vi "Plugin-001-MaterialTest.vi"(0 "Configuration Page":refnum<class "Material-ConfigPage.lvclass">, 11 "error in":errorcluster) -> (15 "error out":errorcluster)   [LabVIEW 2013, in "Material-RunTest.lvclass"]
doc: "DisplayName=\"Deploy Configuration Template\"\nDescription=\"This VI serves as a template page for the Deploy Configuration UI.\""
uses:
  Plugins/Run Material Test/Material-RunTest.lvclass
  Reuse Library/featherweight/Core/Sequencer/FTW-Sequencer.lvclass
  Reuse Library/featherweight/Core/Messaging/Message.Actor/FTW-Message-Actor.lvclass
  Material-ConfigPage.lvclass
  <vilib>/Utility/miscctls.llb/LVPointTypeDef.ctl
  Plugins/Motion Control/Motion-ControlAll.lvclass
  <instrlib>/Keyence LK-G5000/Keyence LK-G5000.lvlib
  Reuse Library/Database API/Database-API.lvclass
  <vilib>/addons/_LabVIEW Style Book/Utilities/Style Book Utilities.lvlib
  <vilib>/ErrorRing/Error Ring.xnode
  <vilib>/Utility/error.llb/Error Cluster From Error Code.vi
panel:
  in  "Find Home Position":bool
  out "Average Thickness Line 3":dbl format="%_5g"
  out "Line 3 test passed?":bool
  out "Line 3 Measurement Graph":dbl[](graph)
  out "Average Thickness Line 2":dbl format="%_5g"
  out "Line 2 test passed?":bool
  out "Line 2 Measurement Graph":dbl[](graph)
  out "Average Thickness Line 1":dbl format="%_5g"
  out "Line 1 test passed?":bool
  out "Line 1 Measurement Graph":dbl[](graph)
  in  "Zero Laser":bool
  in  "Stop Button":bool
  out "Overall Sheet Passed?":bool
  out "Total Average Thickness of Sheet":dbl format="%_6g"
  out "Thickness Measured Real Time":dbl format="%_6g"
  in  "Begin Test":bool
  out "Message Received":string
  # "Settings"
  # "Inputs"
  # "Outputs"
  # "First Plugin"
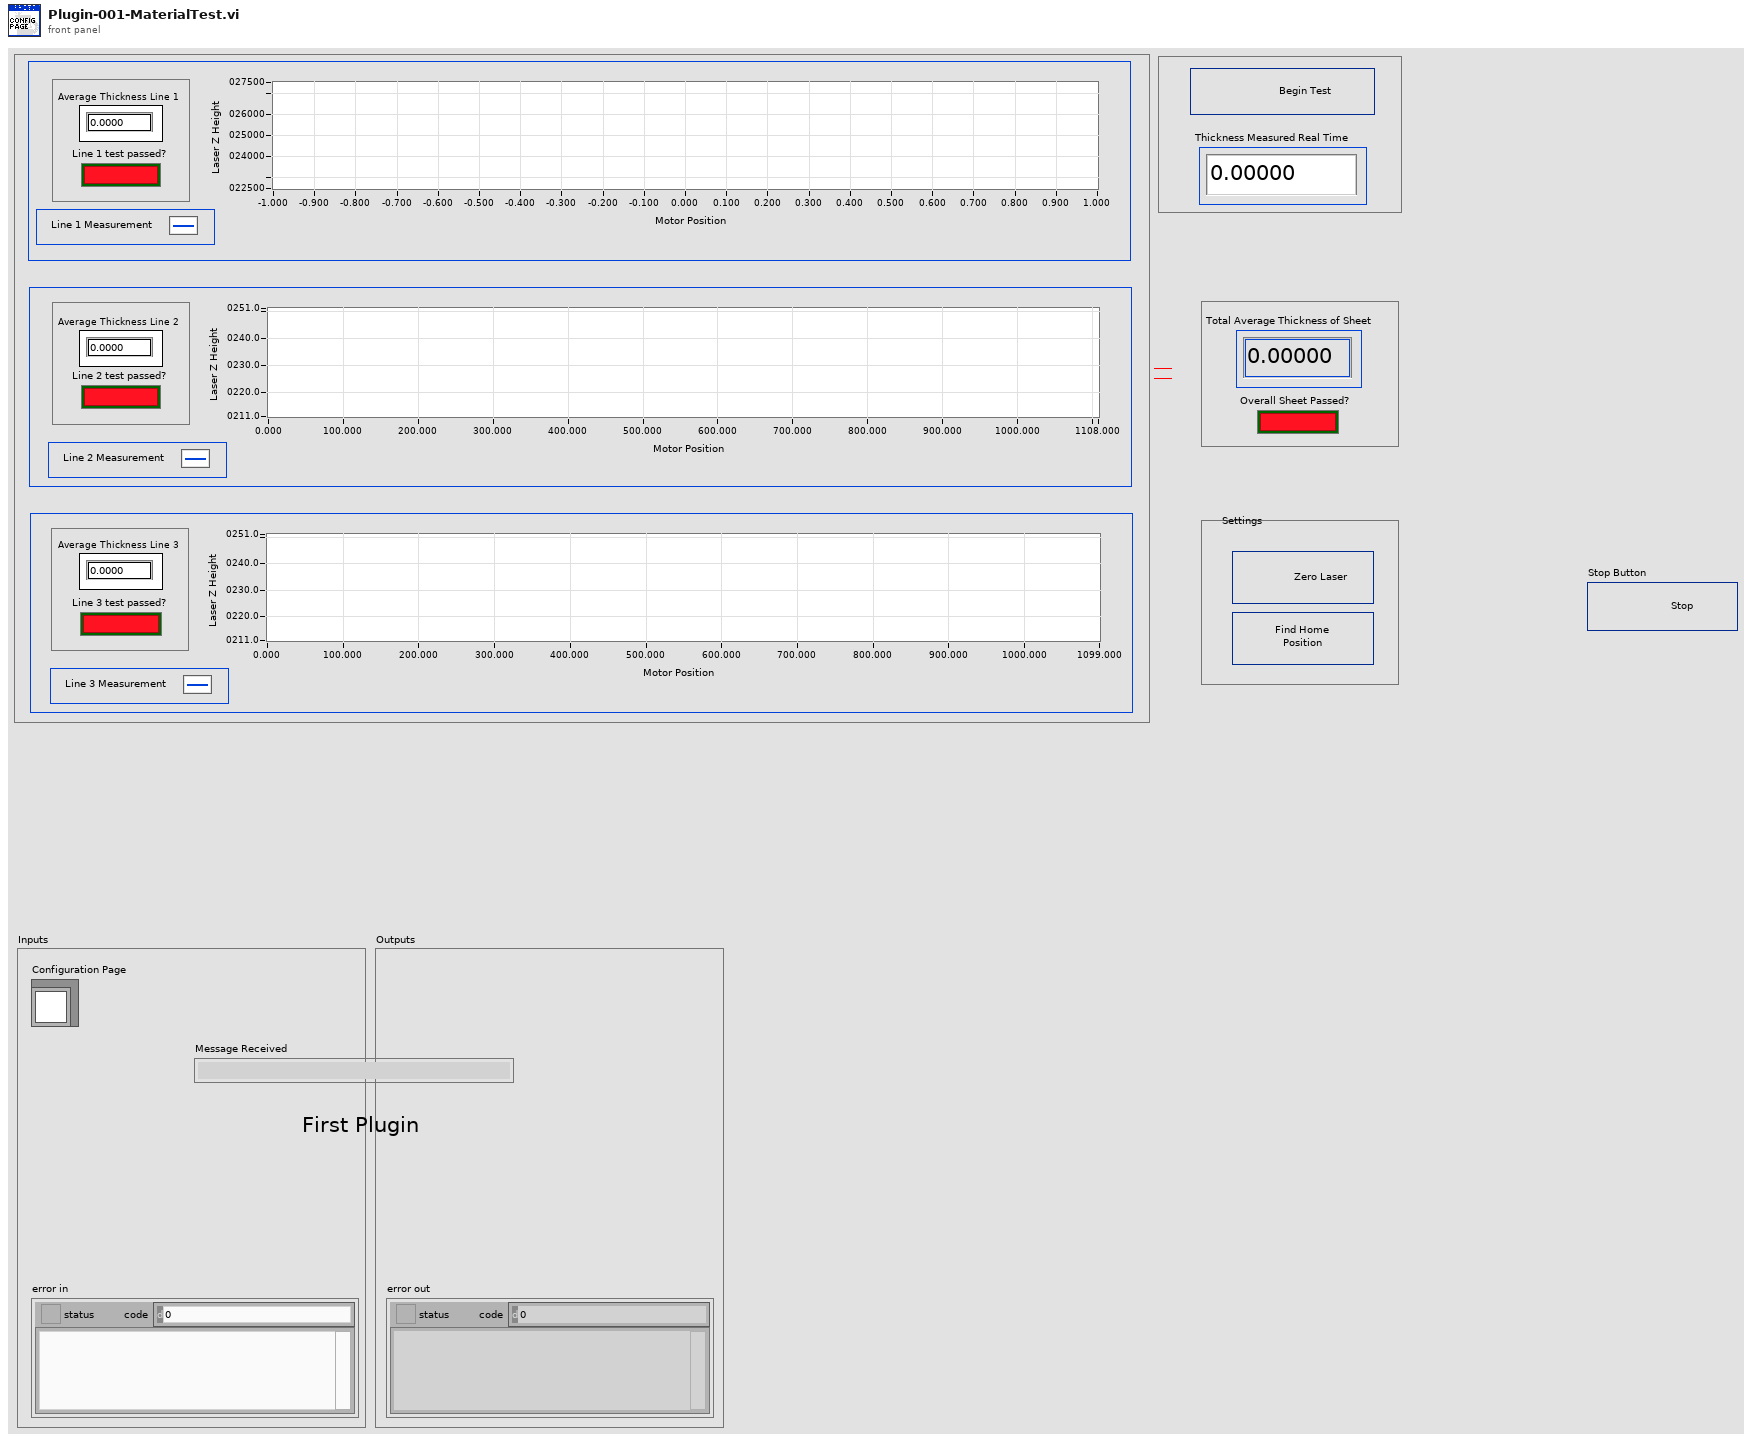
[diagram p1: front panel]
types:
  T1 = enum8{"Enabled", "Disabled", "Disabled and Grayed Out"}
  T2 = typedef "LVPointTypeDef.ctl" = cluster{"Horizontal":i16, "Vertical":i16}
  T3 = cluster{"PageCommands":refnum<event-registration>}
  T4 = cluster{"Zero Button Pressed":bool, "Home Button Pressed":bool}
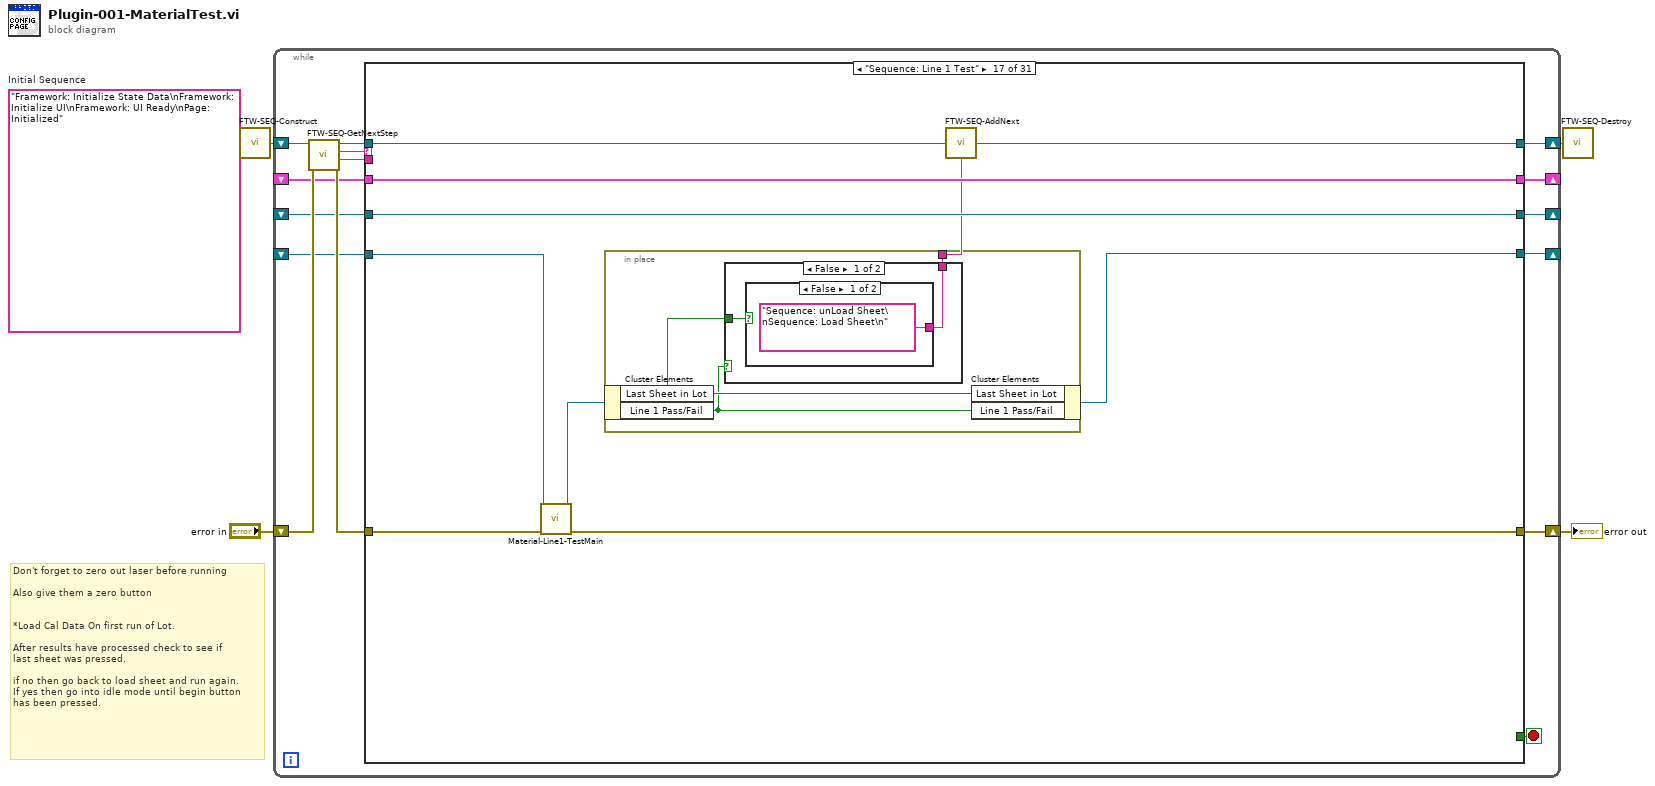
[diagram p0: block diagram]
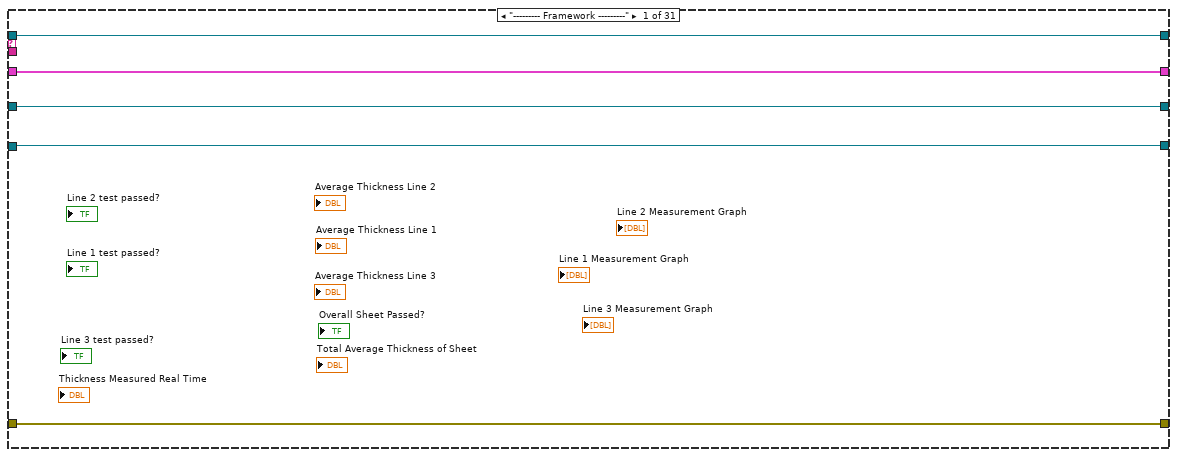
[diagram p2: hidden frame]
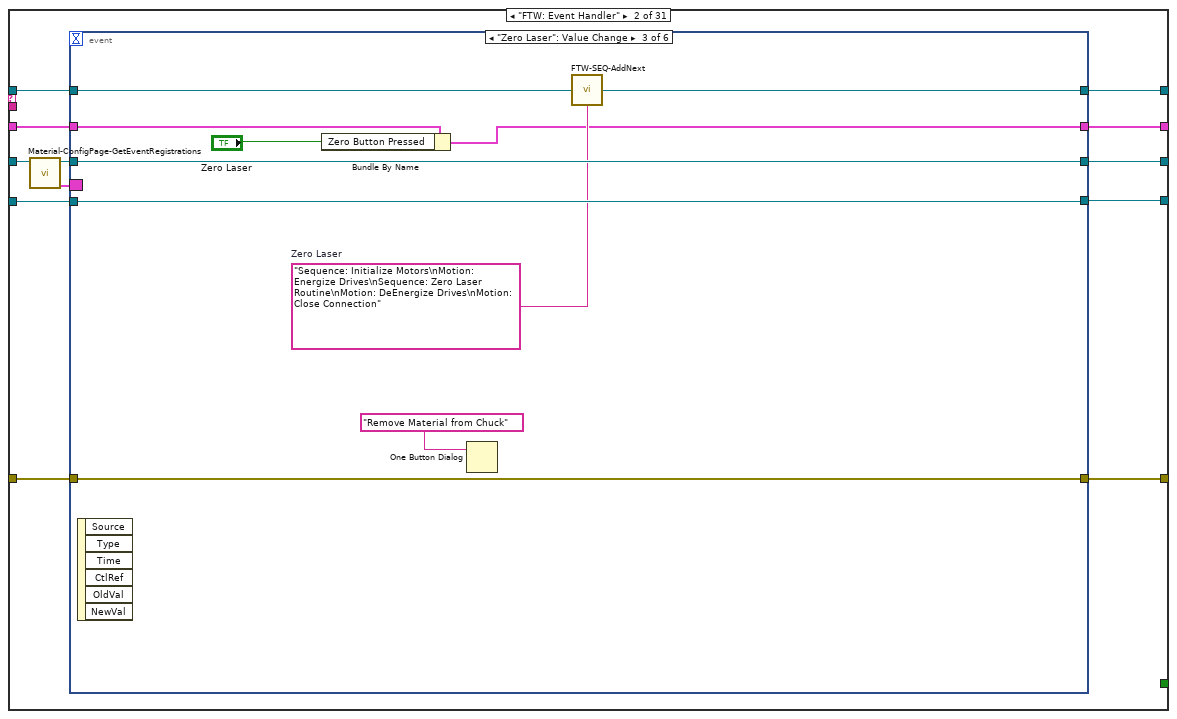
[diagram p3: hidden frame]
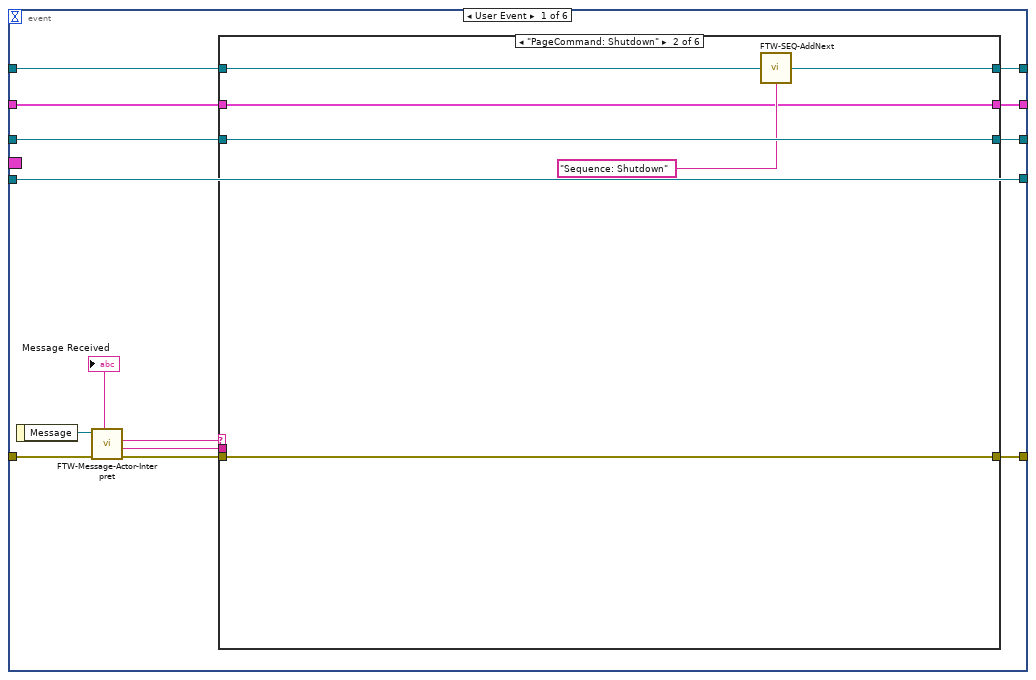
[diagram p4: hidden frame]
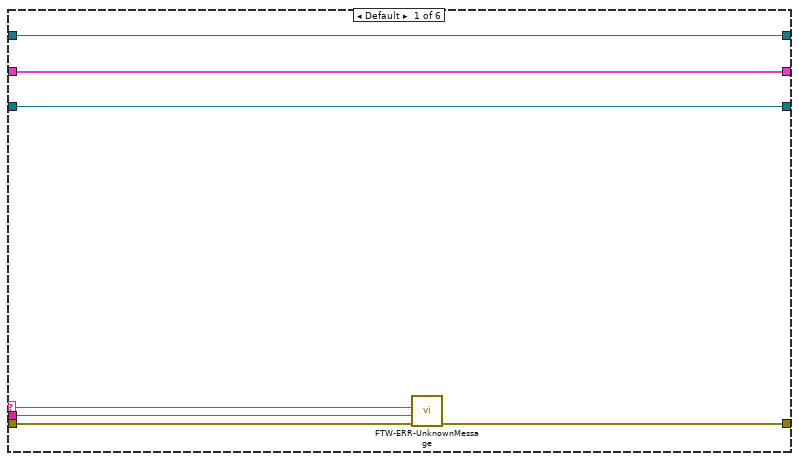
[diagram p5: hidden frame]
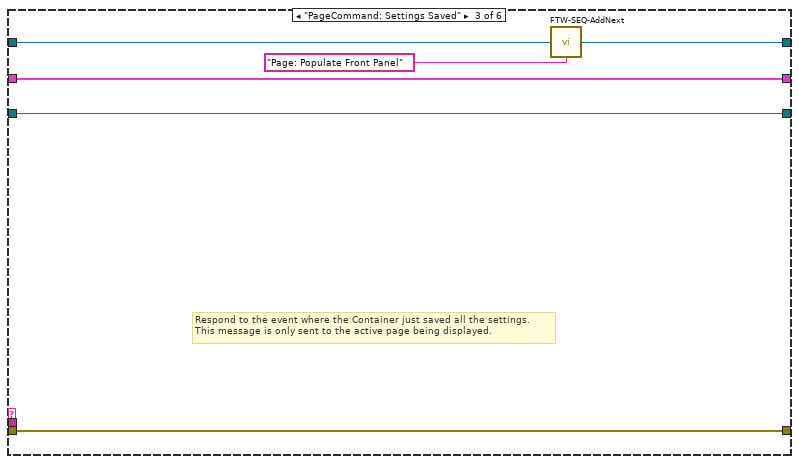
[diagram p6: hidden frame]
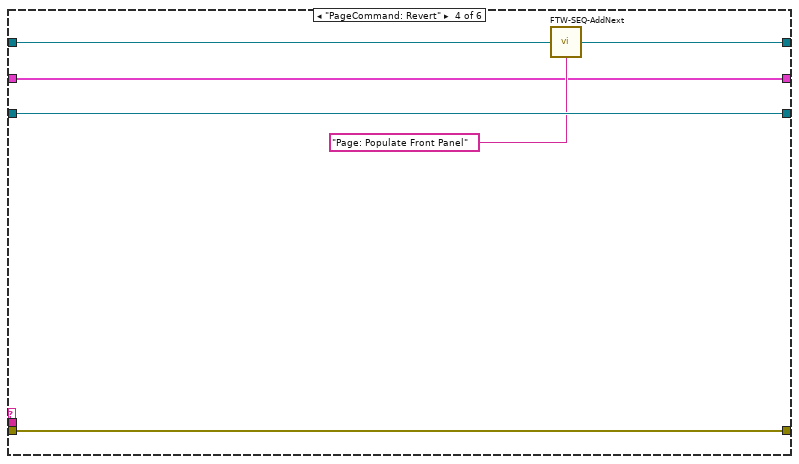
[diagram p7: hidden frame]
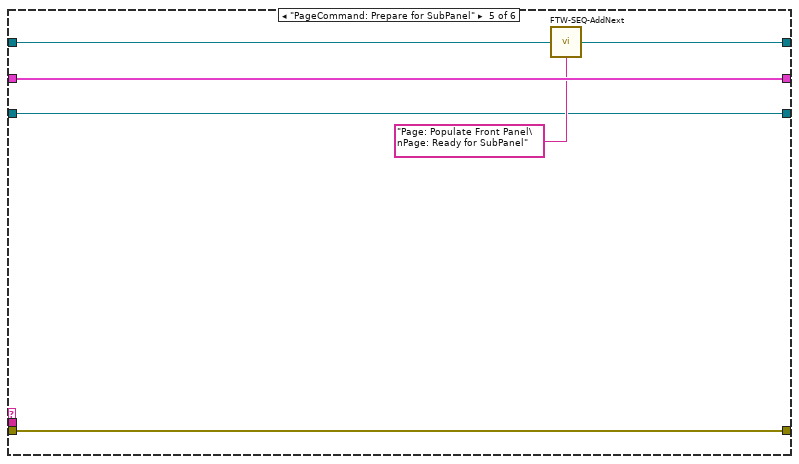
[diagram p8: hidden frame]
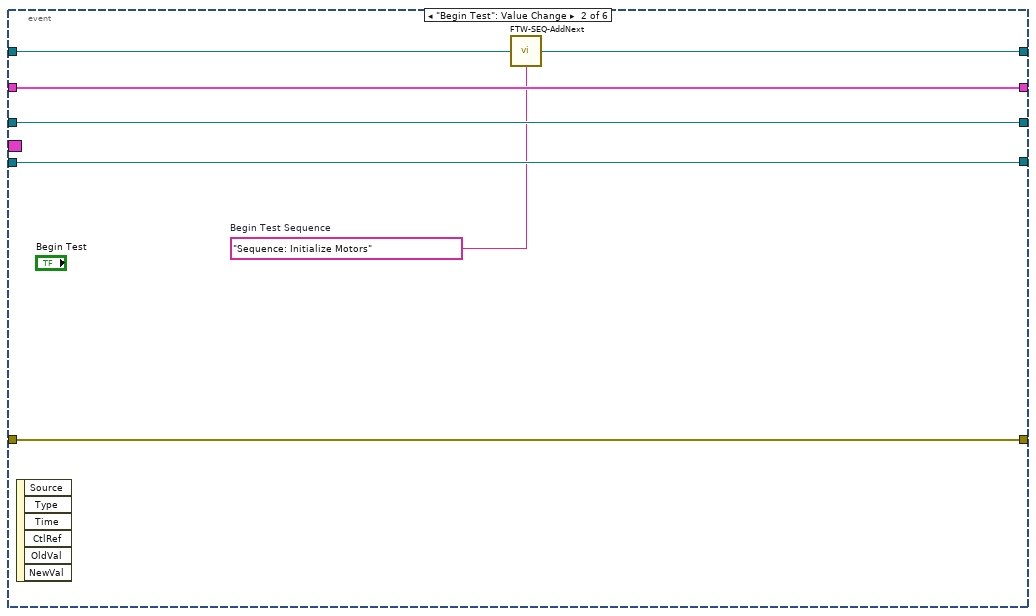
[diagram p10: hidden frame]
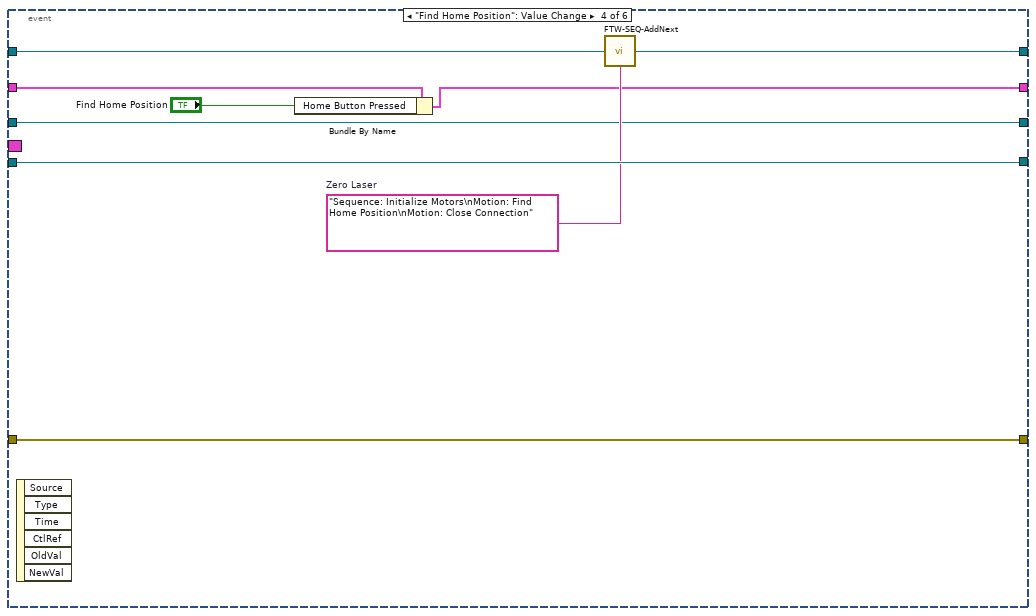
[diagram p11: hidden frame]
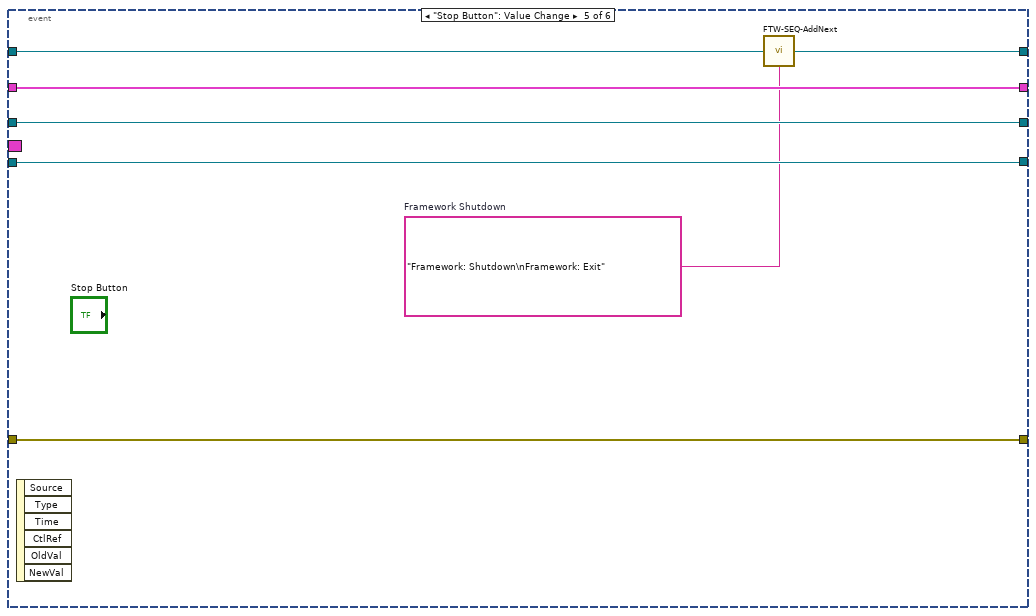
[diagram p12: hidden frame]
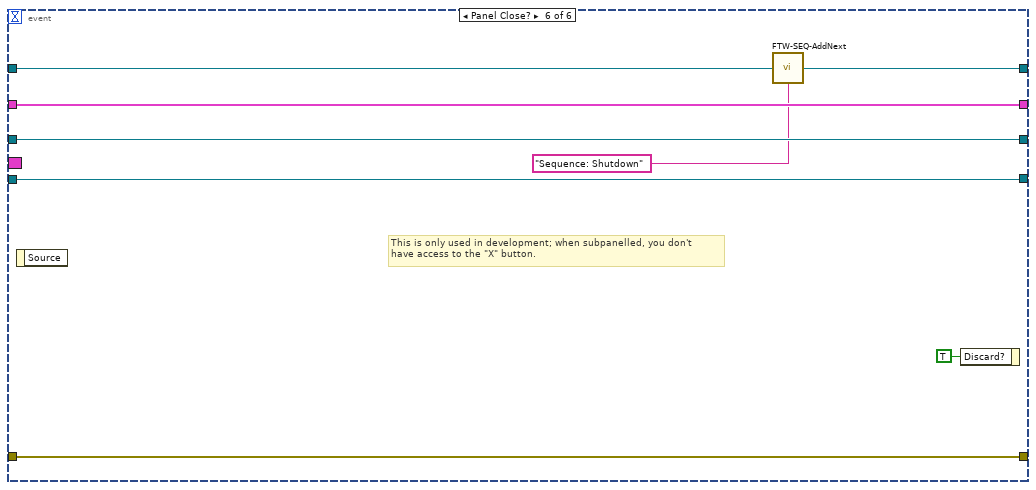
[diagram p13: hidden frame]
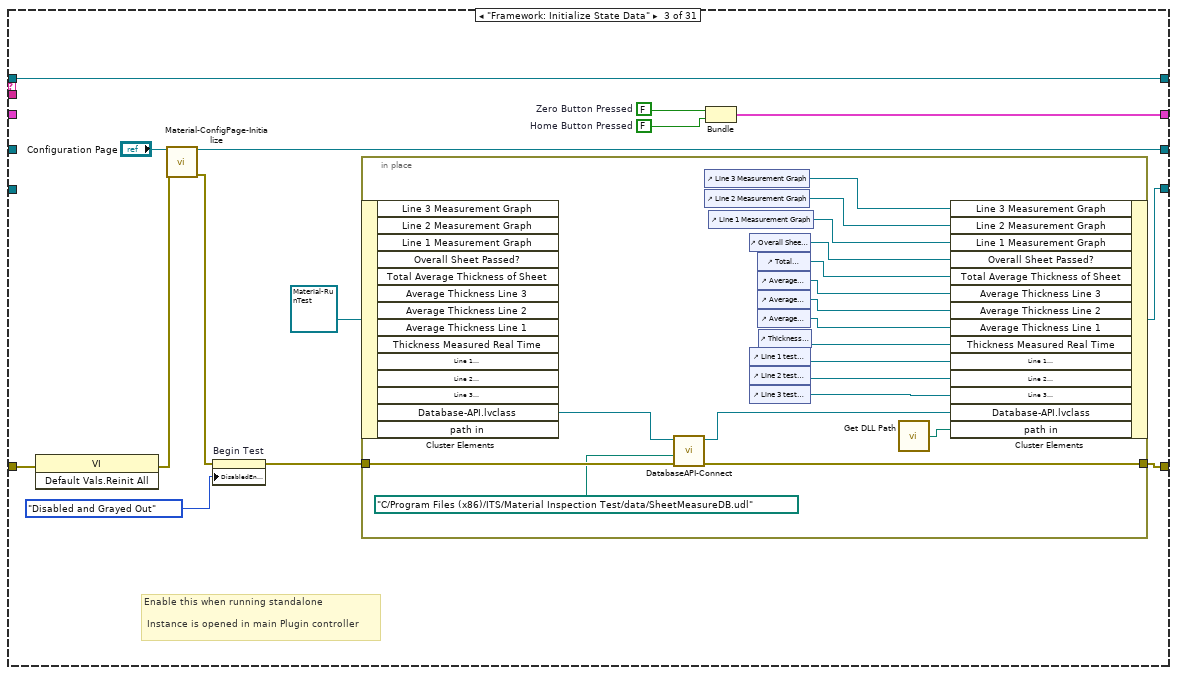
[diagram p14: hidden frame]
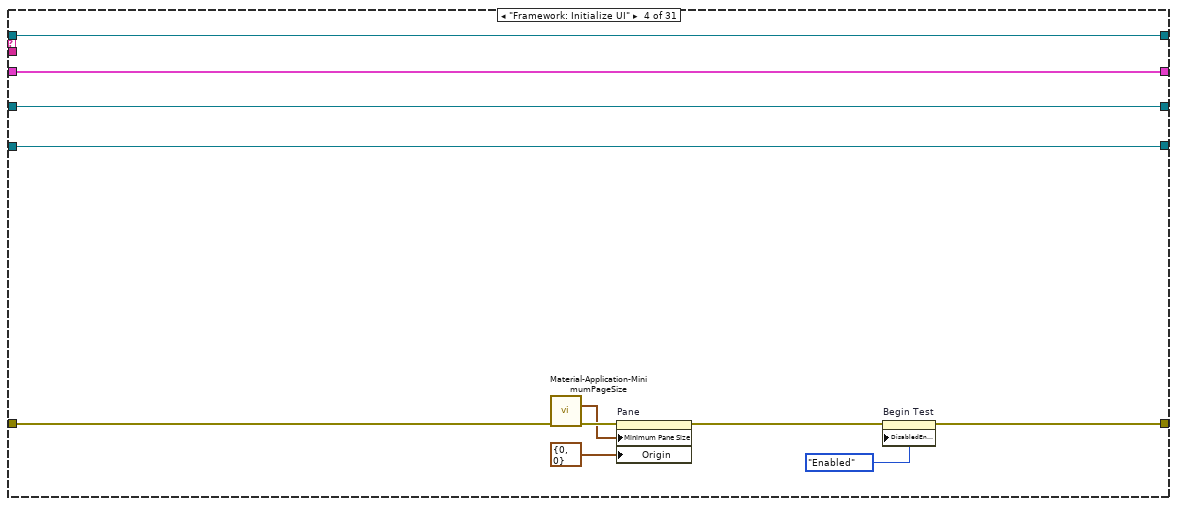
[diagram p15: hidden frame]
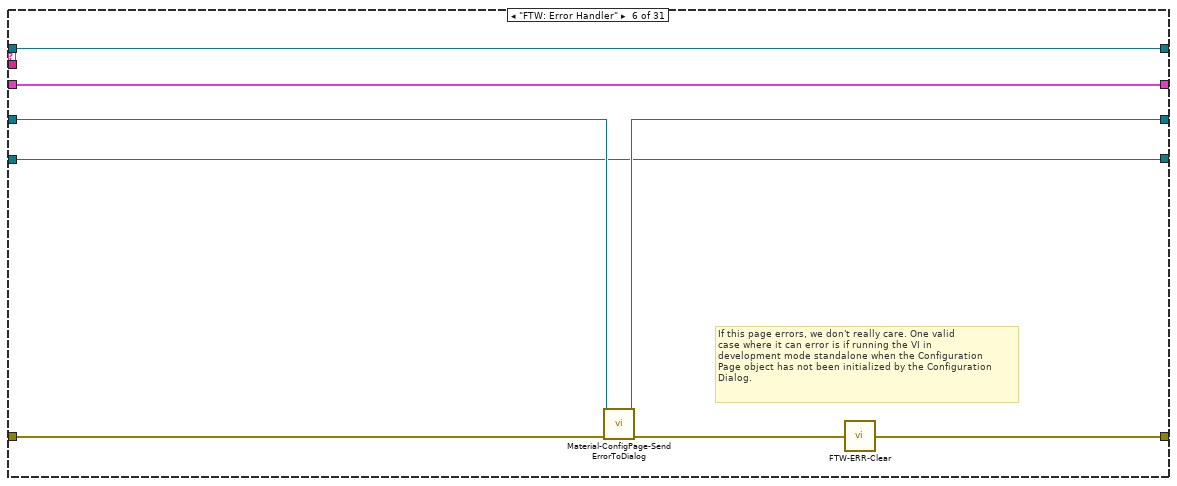
[diagram p17: hidden frame]
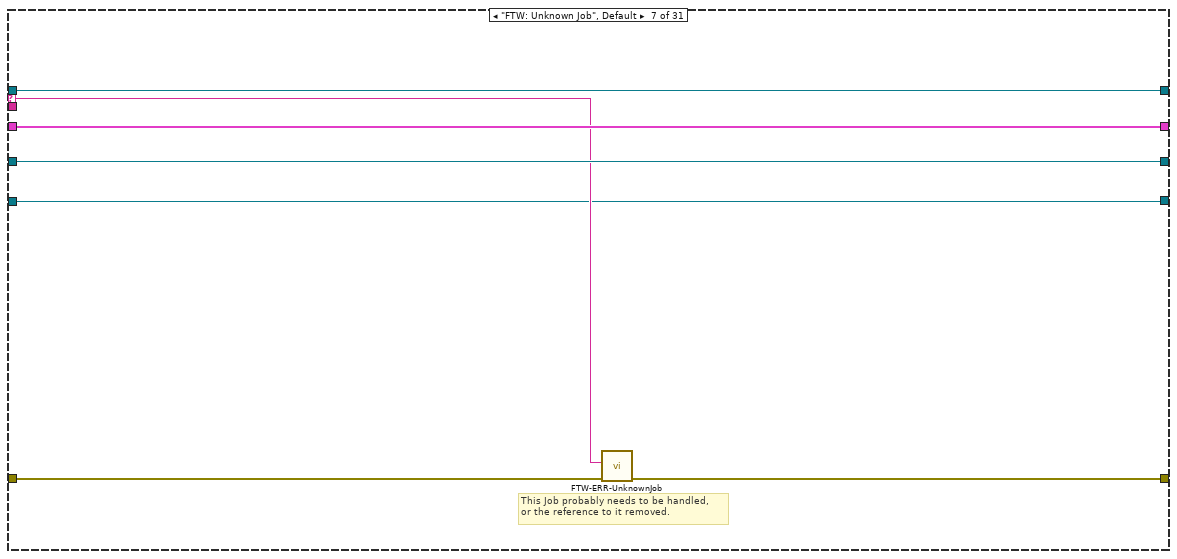
[diagram p18: hidden frame]
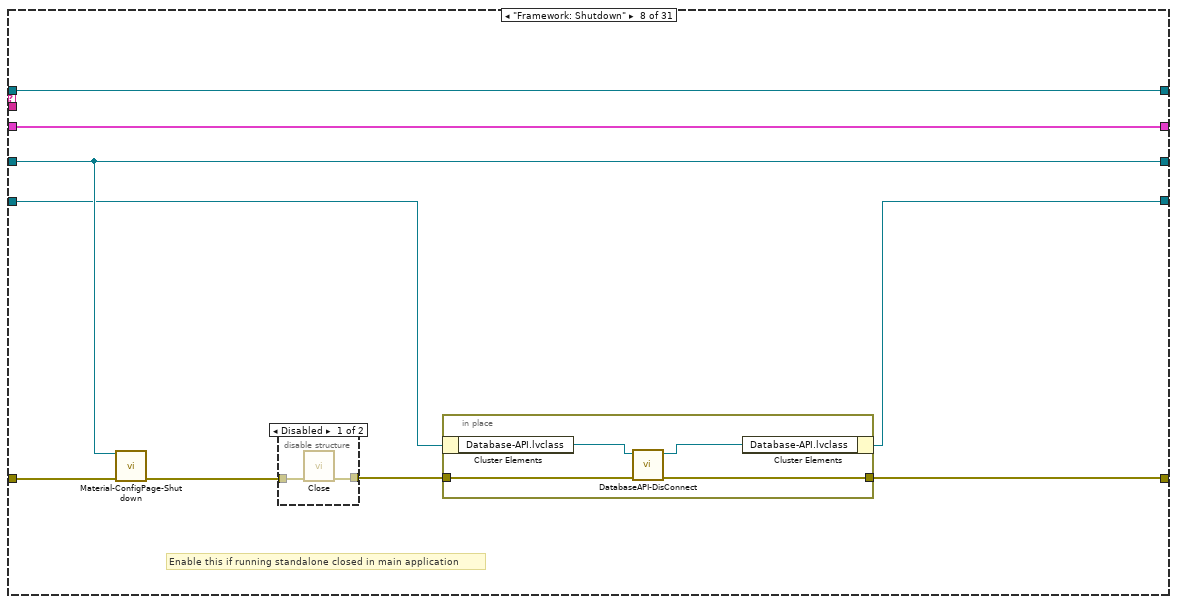
[diagram p19: hidden frame]
diagram:
  w5 = "Framework: Initialize State Data\nFramework: Initialize UI\nFramework: UI Ready\nPage: Initialized"  # Initial Sequence
  # "Don't forget to zero out laser before running\n\nAlso give them a zero button\n\n\n*Load Cal Data On first run of Lot.\n\nAfter results have processed check to see if\nlast sheet was pressed. \n\nif no then go back to load sheet and run again. \nIf yes then go into idle mode until begin button\nhas been pressed."
  n1 = call "FTW-SEQ-Construct.vi"("Initial Sequence"=w5) -> ("Sequencer"=w4:refnum<class "FTW-Sequencer.lvclass">)
  n2 = while {
    shift-right: [w18] -> w3
    shift-left: w4 -> [w9]
    shift-right: [w19] -> w2
    shift-left: "error in" -> [w17]
    shift-right: [w13] -> _
    shift-left: _ -> [w12]
    shift-right: [w11] -> _
    shift-left: _ -> [w10]
    shift-right: [w7] -> _
    shift-left: _ -> [w6]
    stop <- w14 stop-if-true
    n3 = call "FTW-SEQ-GetNextStep.vi"("error in"=w17, "Sequencer"=w9) -> ("error out"=w20:errorcluster, "Job Data"=w8:string, "Current Job"=w15:string, "Sequencer out"=w16:refnum<class "FTW-Sequencer.lvclass">)  [unwired: 6 in]
    n4 = case shown="\"Sequence: Line 1 Test\"" w15 {
      selector: w15 -> [_ _ _ _ _ _ w184 _ _ _ _ _ _ _ _ _ _ _ _ _ _ _ _ _ _ _ _ _ _ _ _]
      tunnel: [w23 w35 w134 w161 w174 w181 w186 w190 w209 w217 w224 w229 w244 w271 w287 w307 w318 w336 w354 w367 w387 w393 w397 w406 w408 w413 w424 w436 w448 w459 w465] -> w19
      tunnel: w20 -> [w23 w34 w137 w159 w174 w178 w187 w196 w209 w217 w224 w236 w249 w274 w286 w306 w320 w338 w356 w376 w387 w394 w397 w407 w408 w416 w427 w440 w451 w459 w472]
      tunnel: w16 -> [w24 w37 w139 w166 w171 w176 w189 w197 w207 w214 w221 w238 w250 w276 w281 w310 w316 w335 w350 w372 w384 w390 w400 w402 w411 w418 w429 w442 w453 w462 w469]
      tunnel: [w24 w36 w139 w166 w171 w176 w189 w197 w207 w213 w220 w237 w250 w275 w283 w310 w314 w334 w349 w373 w384 w390 w400 w402 w411 w418 w429 w442 w453 w462 w468] -> w18
      tunnel: [_ _ _ _ _ _ _ _ TRUE _ _ _ _ _ _ _ _ _ _ _ _ _ _ _ _ _ _ _ _ _ _] -> w14
      tunnel: [w25 w33 w140 w169 w173 w182 w188 w198 w210 w218 w225 w227 w252 w278 w293 w312 w322 w340 w358 w378 w386 w395 w399 w405 w412 w419 w430 w443 w454 w463 w474] -> w13
      tunnel: w12 -> [w25 w31 _ w169 w173 w182 w188 w198 w210 w218 w225 w228 w252 w278 w293 w312 w322 w340 w358 w378 w386 w395 w399 w405 w412 w419 w430 w443 w454 w463 w474]
      tunnel: [w22 w32 w135 w164 w172 w179 w185 w195 w208 w216 w223 w239 w251 w277 w292 w311 w321 w339 w357 w377 w385 w391 w398 w403 w410 w417 w428 w441 w452 w461 w473] -> w11
      tunnel: w10 -> [w22 w30 _ w164 w172 w180 w185 w195 w208 w216 w223 w239 w251 w277 w292 w311 w321 w339 w357 w377 w385 w392 w398 w404 w410 w417 w428 w441 w452 w461 w473]
      tunnel: w8 -> [_ _ _ _ _ _ _ _ _ _ _ _ _ _ _ _ _ _ _ _ _ _ _ _ _ _ _ _ _ _ _]
      tunnel: [w21 w26 w132 w160 w170 w175 w183 w191 w206 w212 w219 w234 w247 w272 w288 w308 w313 w331 w351 w370 w383 w388 w396 w401 w409 w414 w425 w438 w449 w460 w470] -> w7
      tunnel: w6 -> [w21 w27 _ w160 w170 w175 w183 w192 w206 w212 w219 w235 w248 w273 w291 w309 w319 w337 w355 w375 w383 w388 w396 w401 w409 w415 w426 w439 w450 w460 w471]
      frame "--------- Framework ---------" {
      }
      frame "FTW: Event Handler" {
        n5 = call "Material-ConfigPage-GetEventRegistrations.vi"("Configuration Page"=w30) -> ("Events"=w28:T3, "Configuration Page out"=w29:refnum<class "Material-ConfigPage.lvclass">)  [unwired: 9 in]
        n6 = event shown="[2] \"Zero Laser\": Value Change" {
          selector: w28 -> [_ _ _ _ _ _]
          dyn-events: _ -> [_ _ _ _ _ _]
          timeout: _ -> [_ _ _ _ _ _]
          tunnel: w37 -> [w44 w89 w98 w110 w117 w121]
          tunnel: [w45 w88 w97 w109 w118 w120] -> w36
          tunnel: [w49 w86 w102 w106 w112 w124] -> w35
          tunnel: w34 -> [w50 w86 w102 w106 w112 w124]
          tunnel: [w43 w92 w93 w103 w116 w125] -> w33
          tunnel: w31 -> [w42 w92 w94 w104 w116 w125]
          tunnel: w29 -> [w47 w90 w100 w107 w115 w123]
          tunnel: [w46 w90 w100 w107 w115 w123] -> w32
          tunnel: [w38 w91 w101 w111 w114 w119] -> w26
          tunnel: w27 -> [w38 w91 w101 w111 w114 w119]
          event User Event {
            n7 = event-data() -> ("Message"=w40:refnum<class "FTW-Message.lvclass">)  [unwired: 1 in]
            n8 = call "FTW-Message-Actor-Interpret.vi"("error in"=w50, "Message"=w40) -> ("error out"=w48:errorcluster, "Sender"=w39:string, "Parameter"=w41:string)  [unwired: 6 in, 1 out]
            "Message Received" <- w41
            n9 = case shown="\"PageCommand: Shutdown\"" w41 {
              selector: w41 -> [w52 _ _ _ _ _]
              tunnel: [w56 w63 w69 w75 w76 w82] -> w49
              tunnel: w48 -> [w57 w63 w69 w75 w76 w82]
              tunnel: w47 -> [w55 w62 w68 w74 w77 w83]
              tunnel: [w55 w62 w68 w74 w77 w83] -> w46
              tunnel: [w54 w58 w66 w72 w80 w84] -> w45
              tunnel: w44 -> [w54 w61 w67 w73 w81 w84]
              tunnel: [w53 w59 w65 w70 w79 w85] -> w43
              tunnel: w42 -> [w53 w59 w65 w70 w79 w85]
              tunnel: w39 -> [w51 _ _ _ _ _]
              frame Default {
                n10 = call "FTW-ERR-UnknownMessage.vi"("error in"=w57, "Sender"=w51, "Unknown Parameter"=w52) -> ("error out"=w56:errorcluster)  [unwired: 8 in]
              }
              frame "PageCommand: Shutdown" {
                n11 = call "FTW-SEQ-AddNext.vi"("Add Next in Sequence"="Sequence: Shutdown", "Sequencer"=w61) -> ("Sequencer out"=w58:refnum<class "FTW-Sequencer.lvclass">)  [unwired: 2 in]
              }
              frame "PageCommand: Settings Saved" {
                # "Respond to the event where the Container just saved all the settings.\nThis message is only sent to the active page being displayed."
                n12 = call "FTW-SEQ-AddNext.vi"("Add Next in Sequence"="Page: Populate Front Panel" ("Add to Top of Sequence"), "Sequencer"=w67) -> ("Sequencer out"=w66:refnum<class "FTW-Sequencer.lvclass">)  [unwired: 2 in]
              }
              frame "PageCommand: Revert" {
                n13 = call "FTW-SEQ-AddNext.vi"("Add Next in Sequence"="Page: Populate Front Panel", "Sequencer"=w73) -> ("Sequencer out"=w72:refnum<class "FTW-Sequencer.lvclass">)  [unwired: 2 in]
              }
              frame "PageCommand: Prepare for SubPanel" {
                n14 = call "FTW-SEQ-AddNext.vi"("Add Next in Sequence"="Page: Populate Front Panel\nPage: Ready for SubPanel", "Sequencer"=w81) -> ("Sequencer out"=w80:refnum<class "FTW-Sequencer.lvclass">)  [unwired: 2 in]
              }
              frame "PageCommand: Displayed" {
                # "This case is important for dynamically-registering\nVI Server objects for events, since that operation\nwould fail if the Front Panel is not currently being shown.\nThis is because, those references have not yet been constructed."
              }
            }
          }
          event "Begin Test": Value Change {
            w87 = "Sequence: Initialize Motors"  # Begin Test Sequence
            n15 = event-data() -> ()  [unwired: 1 in, 6 out]
            n16 = call "FTW-SEQ-AddNext.vi"("Add Next in Sequence"=w87, "Sequencer"=w89) -> ("Sequencer out"=w88:refnum<class "FTW-Sequencer.lvclass">)  [unwired: 2 in]
          }
          event "Zero Laser": Value Change {
            w99 = "Sequence: Initialize Motors\nMotion: Energize Drives\nSequence: Zero Laser Routine\nMotion: DeEnergize Drives\nMotion: Close Connection"  # Zero Laser
            n17 = event-data() -> ()  [unwired: 1 in, 6 out]
            n18 = Bundle By Name(cluster=w94, "Zero Button Pressed"="Zero Laser") -> (w93:T4)
            n19 = One Button Dialog(message="Remove Material from Chuck") -> ()  [unwired: 1 in, 1 out]
            n20 = call "FTW-SEQ-AddNext.vi"("Add Next in Sequence"=w99, "Sequencer"=w98) -> ("Sequencer out"=w97:refnum<class "FTW-Sequencer.lvclass">)  [unwired: 2 in]
          }
          event "Find Home Position": Value Change {
            w108 = "Sequence: Initialize Motors\nMotion: Find Home Position\nMotion: Close Connection"  # Zero Laser
            n21 = event-data() -> ()  [unwired: 1 in, 6 out]
            n22 = Bundle By Name(cluster=w104, "Home Button Pressed"="Find Home Position") -> (w103:T4)
            n23 = call "FTW-SEQ-AddNext.vi"("Add Next in Sequence"=w108, "Sequencer"=w110) -> ("Sequencer out"=w109:refnum<class "FTW-Sequencer.lvclass">)  [unwired: 2 in]
          }
          event "Stop Button": Value Change {
            w113 = "Framework: Shutdown\nFramework: Exit"  # Framework Shutdown
            n24 = event-data() -> ()  [unwired: 1 in, 6 out]
            n25 = call "FTW-SEQ-AddNext.vi"("Add Next in Sequence"=w113, "Sequencer"=w117) -> ("Sequencer out"=w118:refnum<class "FTW-Sequencer.lvclass">)  [unwired: 2 in]
          }
          event Panel Close? {
            # "This is only used in development; when subpanelled, you don't\nhave access to the \"X\" button."
            n26 = event-data() -> ()  [unwired: 1 in, 1 out]
            n27 = call "FTW-SEQ-AddNext.vi"("Add Next in Sequence"="Sequence: Shutdown" ("Add to Top of Queue"), "Sequencer"=w121) -> ("Sequencer out"=w120:refnum<class "FTW-Sequencer.lvclass">)  [unwired: 2 in]
            n28 = event-data("Discard?"=TRUE) -> ()  [unwired: 1 in, 1 out]
          }
        }
      }
      frame "Framework: Initialize State Data" {
        w128 = FALSE  # Home Button Pressed
        w129 = FALSE  # Zero Button Pressed
        # "Enable this when running standalone\n\n Instance is opened in main Plugin controller"
        n29 = invoke class="VI" method="Default Vals.Reinit All"(error in=w137) -> (error out=w136:errorcluster)  [unwired: 2 in, 2 out]
        n30 = call-dynamic "Material-ConfigPage-Initialize.vi"("Configuration Page"="Configuration Page", "error in"=w136) -> ("Configuration Page out"=w135:refnum<class "Material-ConfigPage.lvclass">, "error out"=w127:errorcluster)  [unwired: 12 in]
        n31 = property on="Begin Test" class="Bool"(error in=w127, "DisabledEnum"=T1."Disabled and Grayed Out" ("Disabled")) -> (error out=w130:errorcluster)  [unwired: 1 in, 1 out]
        n32 = in-place {
          in-place-border: w130 -> [w145]
          in-place-border: [w142] -> w134
          n33 = in-place-cluster #1(refnum<class "Material-RunTest.lvclass"> refnum ("Material-RunTest.lvclass")) -> ("Database-API.lvclass"=w146:refnum<class "Database-API.lvclass">)  [unwired: 13 out]
          n34 = call "DatabaseAPI-Connect.vi"("error in (no error)"=w145, "Database (mdb)  File Path"=path "C:/Program Files (x86)/ITS/Material Inspection Test/data/SheetMeasureDB.udl", "Database-API in"=w146) -> ("error out"=w142:errorcluster, "Database-API out"=w149:refnum<class "Database-API.lvclass">)  [unwired: 7 in]
          n35 = control-ref of="Line 3 Measurement Graph"() -> (w147:refnum<vi>)
          n36 = control-ref of="Line 2 Measurement Graph"() -> (w148:refnum<vi>)
          n37 = control-ref of="Line 1 Measurement Graph"() -> (w144:refnum<vi>)
          n38 = control-ref of="Overall Sheet Passed?"() -> (w150:refnum<vi>)
          n39 = control-ref of="Line 1 test passed?"() -> (w157:refnum<vi>)
          n40 = control-ref of="Line 2 test passed?"() -> (w156:refnum<vi>)
          n41 = control-ref of="Line 3 test passed?"() -> (w155:refnum<vi>)
          n42 = control-ref of="Total Average Thickness of Sheet"() -> (w151:refnum<vi>)
          n43 = control-ref of="Average Thickness Line 3"() -> (w152:refnum<vi>)
          n44 = control-ref of="Average Thickness Line 2"() -> (w153:refnum<vi>)
          n45 = control-ref of="Average Thickness Line 1"() -> (w154:refnum<vi>)
          n46 = control-ref of="Thickness Measured Real Time"() -> (w158:refnum<vi>)
          n47 = call <instrlib>:"Get DLL Path.vi"() -> ("DLL Path"=w143:path)  [unwired: 1 in]
          n48 = in-place-cluster #1("Line 3 Measurement Graph"=w147, "Line 2 Measurement Graph"=w148, "Line 1 Measurement Graph"=w144, "Overall Sheet Passed?"=w150, "Total Average Thickness of Sheet"=w151, "Average Thickness Line 3"=w152, "Average Thickness Line 2"=w153, "Average Thickness Line 1"=w154, "Thickness Measured Real Time"=w158, "Line 1\ntest passed?"=w157, "Line 2\ntest passed?"=w156, "Line 3\ntest passed?"=w155, "Database-API.lvclass"=w149, "path in"=w143) -> (w132:refnum<class "Material-RunTest.lvclass">)
        }
        n49 = Bundle("Zero Button Pressed"=w129, "Home Button Pressed"=w128) -> (w140:T4)  [unwired: 1 in]
      }
      frame "Framework: Initialize UI" {
        n50 = call "Material-Application-MinimumPageSize.vi"("error in"=w159) -> ("Minimum Pane Size"=w167:cluster{"Horizontal":i16, "Vertical":i16}, "error out"=w168:errorcluster)  [unwired: 13 in]
        n51 = property on="Pane" class="Pane"(error in=w168, "Minimum Pane Size"=w167, "Origin"=T2 {"Horizontal"=0, "Vertical"=0}) -> (error out=w163:errorcluster)  [unwired: 1 in, 1 out]
        n52 = property on="Begin Test" class="Bool"(error in=w163, "DisabledEnum"=T1."Enabled" ("Disabled")) -> (error out=w161:errorcluster)  [unwired: 1 in, 1 out]
      }
      frame "Framework: UI Ready" {
      }
      frame "FTW: Error Handler" {
        # "If this page errors, we don't really care. One valid\ncase where it can error is if running the VI in\ndevelopment mode standalone when the Configuration\nPage object has not been initialized by the Configuration\nDialog."
        n53 = call "Material-ConfigPage-SendErrorToDialog.vi"("Configuration Page in"=w180, "error in"=w178) -> ("Configuration Page out"=w179:refnum<class "Material-ConfigPage.lvclass">, "error out"=w177:errorcluster)  [unwired: 12 in]
        n54 = call "FTW-ERR-Clear.vi"("error to snuff"=w177) -> ("no error"=w181:errorcluster)
      }
      frame "FTW: Unknown Job", Default {
        # "This Job probably needs to be handled,\nor the reference to it removed."
        n55 = call "FTW-ERR-UnknownJob.vi"("error in"=w187, "Unknown Job"=w184) -> ("error out"=w186:errorcluster)  [unwired: 9 in]
      }
      frame "Framework: Shutdown" {
        # "Enable this if running standalone closed in main application"
        n56 = call "Material-ConfigPage-Shutdown.vi"("Configuration Page"=w195, "error in"=w196) -> ("error out"=w194:errorcluster)  [unwired: 13 in]
        n57 = disable-structure shown="Disabled" {
          disable-tunnel: w194 -> [w204 w205]
          disable-tunnel: [w203 w205] -> w193
          frame Disabled {
            n58 = call <instrlib>:"Close.vi"("error in (no error)"=w204) -> ("error out"=w203:errorcluster)  [unwired: 10 in]
          }
          frame Enabled {
          }
        }
        n59 = in-place {
          in-place-border: w193 -> [w200]
          in-place-border: [w199] -> w190
          n60 = in-place-cluster #2(w192) -> ("Database-API.lvclass"=w202:refnum<class "Database-API.lvclass">)
          n61 = call "DatabaseAPI-DisConnect.vi"("error in (no error)"=w200, "Database-API in"=w202) -> ("error out"=w199:errorcluster, "Database-API out"=w201:refnum<class "Database-API.lvclass">)  [unwired: 8 in]
          n62 = in-place-cluster #2("Database-API.lvclass"=w201) -> (w191:refnum<class "Material-RunTest.lvclass">)
        }
      }
      frame "Framework: Exit" {
        # "This is the last frame to execute;\ntypically, no code is placed in this\ncase -- anything that needs to be\nhandled prior to exiting this VI is\nperformed in another Step."
      }
      frame "--------- Sequences ---------" {
        w215 = ""  # Add to Top of Sequence
        n63 = call "FTW-SEQ-AddNext.vi"("Add Next in Sequence"=w215, "Sequencer"=w214) -> ("Sequencer out"=w213:refnum<class "FTW-Sequencer.lvclass">)  [unwired: 2 in]
      }
      frame "Sequence: Shutdown" {
        w222 = "Framework: Shutdown\nFramework: Exit"  # Framework Shutdown
        n64 = call "FTW-SEQ-AddNext.vi"("Add Next in Sequence"=w222, "Sequencer"=w221) -> ("Sequencer out"=w220:refnum<class "FTW-Sequencer.lvclass">)  [unwired: 2 in]
      }
      frame "Sequence: Initialize Motors" {
        n65 = in-place {
          in-place-border: w236 -> [w242]
          in-place-border: [w241] -> w230
          n66 = in-place-cluster #3(w235) -> ("Motion-ControlAll.lvclass"=w243:refnum<class "Motion-ControlAll.lvclass">)
          n67 = call "Motion-Intialize-Drives.vi"("error in (no error)"=w242, "Motion-ControlAll in"=w243) -> ("error out"=w241:errorcluster, "Motion-ControlAll out"=w240:refnum<class "Motion-ControlAll.lvclass">)  [unwired: 8 in]
          n68 = in-place-cluster #3("Motion-ControlAll.lvclass"=w240) -> (w234:refnum<class "Material-RunTest.lvclass">)
        }
        n69 = Unbundle By Name(w230) -> ("status"=w233:bool)
        n70 = Equal?(x=TRUE, y=w233) -> (x = y?=w231:bool)
        n71 = call "Material-SettingsButtonPressed.vi"("error in (no error)"=w230, "Boolean"=w231, "Cluster in"=w228) -> ("error out"=w229:errorcluster, "Cluster out"=w227:T4, "Begin Test Sequence"=w226:string)  [unwired: 6 in]
        n72 = call "FTW-SEQ-AddNext.vi"("Add Next in Sequence"=w226, "Sequencer"=w238) -> ("Sequencer out"=w237:refnum<class "FTW-Sequencer.lvclass">)  [unwired: 2 in]
      }
      frame "Sequence: Zero Laser Routine" {
        n73 = in-place {
          in-place-border: w249 -> [w266]
          in-place-border: [w257] -> w246
          n74 = in-place-cluster #4(w248) -> ("Motion-ControlAll.lvclass"=w265:refnum<class "Motion-ControlAll.lvclass">)
          n75 = call "Motion-Move-XandY.vi"("Y Drive Acc/Speed/Velocity"="MA1: A 10: V 20: AD 10: D ", "X Drive Acc/Speed/Velocity"="MA1: A 10: V 20: AD 10: D ", "error in (no error)"=w266, "X Coordinates"="0", "Y Coordinates"="200000", "Motion-ControlAll in"=w265) -> ("error out"=w263:errorcluster, "Motion-ControlAll out"=w264:refnum<class "Motion-ControlAll.lvclass">)  [unwired: 4 in]
          n76 = call "Motion-PollAxis-Main.vi"("error in (no error)"=w263, "Motion-ControlAll in"=w264) -> ("error out"=w256:errorcluster, "Motion-ControlAll out"=w262:refnum<class "Motion-ControlAll.lvclass">)  [unwired: 8 in]
          n77 = call <vilib>:"Wait n mSec.vi"("error in (no error)"=w256, "Milliseconds to Wait (500)"=u32 1000) -> ("error out"=w255:errorcluster)  [unwired: 13 in]
          n78 = in-place-cluster #4("Motion-ControlAll.lvclass"=w262) -> (w247:refnum<class "Material-RunTest.lvclass">)
          n79 = call <instrlib>:"LKIF2_SetZero.vi"("error in (no error)"=w255, "OnOff"=TRUE) -> ("error out"=w257:errorcluster)  [unwired: 9 in]
        }
        n80 = property on="Zero Laser" class="Bool (strict)"(error in=w246, "Value"=FALSE ("Zero Laser")) -> (error out=w244:errorcluster)  [unwired: 1 in, 1 out]
      }
      frame "Sequence: Choose Part Number" {
        # "Laser: Change Sampling Rate"
        n81 = call "Material-ChoosePart#-Spec.vi"("error in (no error)"=w274, "Material-RunTest.lvclass"=w273) -> ("error out"=w271:errorcluster, "Cancel Test"=w269:bool, "Invalid Spec Values"=w270:bool, "Material-RunTest.lvclass out"=w272:refnum<class "Material-RunTest.lvclass">)  [unwired: 6 in]
        n82 = Or(x=w270, y=w269) -> (x .or. y?=w267:bool)
        n83 = case shown="False" w267 {
          tunnel: ["Motion: Energize Drives\nSequence: Zero Laser Routine\nSequence: Load Sheet\n\n\n" ("Add Next in Sequence") "" ("Add Next in Sequence")] -> w268
          frame False {
          }
          frame True {
          }
        }
        n84 = call "FTW-SEQ-AddNext.vi"("Add Next in Sequence"=w268, "Sequencer"=w276) -> ("Sequencer out"=w275:refnum<class "FTW-Sequencer.lvclass">)  [unwired: 2 in]
      }
      frame "Sequence: Load Sheet" {
        n85 = invoke class="VI" method="Default Vals.Reinit All"(error in=w286) -> (error out=w285:errorcluster)  [unwired: 2 in, 2 out]
        n86 = in-place {
          in-place-border: w285 -> [w305]
          in-place-border: [w296] -> w290
          n87 = in-place-cluster #5(w291) -> ("Motion-ControlAll.lvclass"=w304:refnum<class "Motion-ControlAll.lvclass">)
          n88 = call "Motion-Move-XandY.vi"("Y Drive Acc/Speed/Velocity"="MA1: A 10: V 20: AD 10: D ", "X Drive Acc/Speed/Velocity"="MA1: A 10: V 20: AD 10: D ", "error in (no error)"=w305, "X Coordinates"="-880000", "Y Coordinates"="880000", "Motion-ControlAll in"=w304) -> ("error out"=w302:errorcluster, "Motion-ControlAll out"=w303:refnum<class "Motion-ControlAll.lvclass">)  [unwired: 4 in]
          n89 = call "Motion-PollAxis-Main.vi"("error in (no error)"=w302, "Motion-ControlAll in"=w303) -> ("error out"=w296:errorcluster, "Motion-ControlAll out"=w301:refnum<class "Motion-ControlAll.lvclass">)  [unwired: 8 in]
          n90 = in-place-cluster #5("Motion-ControlAll.lvclass"=w301) -> (w289:refnum<class "Material-RunTest.lvclass">)
        }
        n91 = call "Material-LoadSheet-Dialog.vi"("error in"=w290, "Material-RunTest.lvclass in"=w289) -> ("error out"=w287:errorcluster, "Cancel Test"=w284:bool, "Material-RunTest.lvclass out"=w288:refnum<class "Material-RunTest.lvclass">)  [unwired: 7 in]
        n92 = case shown="False" w284 {
          tunnel: ["Sequence: Line 1 Test\n\n" ("Add Next in Sequence") "Motion: DeEnergize Drives\nMotion: Close Connection" ("Add Next in Sequence")] -> w282
          frame False {
          }
          frame True {
          }
        }
        n93 = call "FTW-SEQ-AddNext.vi"("Add Next in Sequence"=w282, "Sequencer"=w281) -> ("Sequencer out"=w283:refnum<class "FTW-Sequencer.lvclass">)  [unwired: 2 in]
      }
      frame "Sequence: unLoad Sheet" {
        n94 = call "Material-UnLoad-ResultCheck.vi"("error in (no error)"=w306, "Material-RunTest in"=w309) -> ("error out"=w307:errorcluster, "Material-RunTest out"=w308:refnum<class "Material-RunTest.lvclass">)  [unwired: 8 in]
      }
      frame "Sequence: Line 1 Test" {
        n95 = call "Material-Line1-TestMain.vi"("error in (no error)"=w320, "Material-RunTest in"=w319) -> ("error out"=w318:errorcluster, "Material-RunTest out"=w317:refnum<class "Material-RunTest.lvclass">)  [unwired: 8 in]
        n96 = in-place {
          in-place-border: [w325] -> w315
          n97 = in-place-cluster #6(w317) -> ("Last Sheet in Lot"=w324:bool, "Line 1 Pass/Fail"=w323:bool)
          n98 = case shown="False" w323 {
            tunnel: [w327 "Sequence: Line 2 Test" ("Add Next in Sequence")] -> w325
            tunnel: w324 -> [w326 _]
            frame False {
              n99 = case shown="False" w326 {
                tunnel: ["Sequence: unLoad Sheet\nSequence: Load Sheet\n" ("Add Next in Sequence") "Sequence: unLoad Sheet\nMotion: DeEnergize Drives\nMotion: Close Connection" ("Add Next in Sequence")] -> w327
                frame False {
                }
                frame True {
                }
              }
            }
            frame True {
            }
          }
          n100 = in-place-cluster #6("Last Sheet in Lot"=w324, "Line 1 Pass/Fail"=w323) -> (w313:refnum<class "Material-RunTest.lvclass">)
        }
        n101 = call "FTW-SEQ-AddNext.vi"("Add Next in Sequence"=w315, "Sequencer"=w316) -> ("Sequencer out"=w314:refnum<class "FTW-Sequencer.lvclass">)  [unwired: 2 in]
      }
      frame "Sequence: Line 2 Test" {
        n102 = call "Material-Line2-TestMain.vi"("error in (no error)"=w338, "Material-RunTest in"=w337) -> ("error out"=w336:errorcluster, "Material-RunTest out"=w332:refnum<class "Material-RunTest.lvclass">)  [unwired: 8 in]
        n103 = in-place {
          in-place-border: [w343] -> w333
          n104 = in-place-cluster #7(w332) -> ("Last Sheet in Lot"=w342:bool, "Line 2 Pass/Fail"=w341:bool)
          n105 = case shown="False" w341 {
            tunnel: [w345 "Sequence: Line 3 Test" ("Add Next in Sequence")] -> w343
            tunnel: w342 -> [w344 _]
            frame False {
              n106 = case shown="False" w344 {
                tunnel: ["Sequence: unLoad Sheet\nSequence: Load Sheet\n" ("Add Next in Sequence") "Sequence: unLoad Sheet\nMotion: DeEnergize Drives\nMotion: Close Connection" ("Add Next in Sequence")] -> w345
                frame False {
                }
                frame True {
                }
              }
            }
            frame True {
            }
          }
          n107 = in-place-cluster #7("Last Sheet in Lot"=w342, "Line 2 Pass/Fail"=w341) -> (w331:refnum<class "Material-RunTest.lvclass">)
        }
        n108 = call "FTW-SEQ-AddNext.vi"("Add Next in Sequence"=w333, "Sequencer"=w335) -> ("Sequencer out"=w334:refnum<class "FTW-Sequencer.lvclass">)  [unwired: 2 in]
      }
      frame "Sequence: Line 3 Test" {
        n109 = call "Material-Line3-TestMain.vi"("error in (no error)"=w356, "Material-RunTest in"=w355) -> ("error out"=w354:errorcluster, "Material-RunTest out"=w352:refnum<class "Material-RunTest.lvclass">)  [unwired: 8 in]
        n110 = in-place {
          in-place-border: [w361] -> w353
          n111 = in-place-cluster #8(w352) -> ("Last Sheet in Lot"=w360:bool, "Line 3 Pass/Fail"=w359:bool)
          n112 = case shown="False" w359 {
            tunnel: [w363 "Sequence: Process Results" ("Add Next in Sequence")] -> w361
            tunnel: w360 -> [w362 _]
            frame False {
              n113 = case shown="False" w362 {
                tunnel: ["Sequence: unLoad Sheet\nSequence: Load Sheet\n" ("Add Next in Sequence") "Sequence: unLoad Sheet\nMotion: DeEnergize Drives\nMotion: Close Connection" ("Add Next in Sequence")] -> w363
                frame False {
                }
                frame True {
                }
              }
            }
            frame True {
            }
          }
          n114 = in-place-cluster #8("Last Sheet in Lot"=w360, "Line 3 Pass/Fail"=w359) -> (w351:refnum<class "Material-RunTest.lvclass">)
        }
        n115 = call "FTW-SEQ-AddNext.vi"("Add Next in Sequence"=w353, "Sequencer"=w350) -> ("Sequencer out"=w349:refnum<class "FTW-Sequencer.lvclass">)  [unwired: 2 in]
      }
      frame "Sequence: Process Results" {
        n116 = call "Material-ProcessResults.vi"("error in (no error)"=w376, "Material-RunTest in"=w375) -> ("error out"=w369:errorcluster, "Material-RunTest out"=w374:refnum<class "Material-RunTest.lvclass">)  [unwired: 8 in]
        n117 = call <vilib>:"Wait n mSec.vi"("error in (no error)"=w369, "Milliseconds to Wait (500)"=u32 3000) -> ("error out"=w367:errorcluster)  [unwired: 13 in]
        n118 = in-place {
          in-place-border: [w380] -> w371
          n119 = in-place-cluster #9(w374) -> ("Last Sheet in Lot"=w379:bool)
          n120 = case shown="False" w379 {
            tunnel: ["Sequence: unLoad Sheet\nSequence: Load Sheet\n" ("Add Next in Sequence") "Sequence: unLoad Sheet\nMotion: DeEnergize Drives\nMotion: Close Connection" ("Add Next in Sequence")] -> w380
            frame False {
            }
            frame True {
              # "Unload the sheet: the test\nis finished for specified lot"
            }
          }
          n121 = in-place-cluster #9("Last Sheet in Lot"=w379) -> (w370:refnum<class "Material-RunTest.lvclass">)
        }
        n122 = call "FTW-SEQ-AddNext.vi"("Add Next in Sequence"=w371, "Sequencer"=w372) -> ("Sequencer out"=w373:refnum<class "FTW-Sequencer.lvclass">)  [unwired: 2 in]
      }
      frame "--------- Application Logic ---------" {
      }
      frame "Page: Initialized" {
        w389 = TRUE  # Allow user to open Diagram from SubPanel?
        n123 = call "Material-ConfigPage-Initialized.vi"("Configuration Page"=w392, "Allow user to open Diagram from SubPanel?"=w389, "error in"=w394) -> ("Configuration Page out"=w391:refnum<class "Material-ConfigPage.lvclass">, "error out"=w393:errorcluster)  [unwired: 11 in]
      }
      frame "Page: Populate Front Panel" {
      }
      frame "Page: Ready for SubPanel" {
        n124 = call "Material-ConfigPage-ReadyForSubPanel.vi"("Configuration Page"=w404, "error in"=w407) -> ("Configuration Page out"=w403:refnum<class "Material-ConfigPage.lvclass">, "error out"=w406:errorcluster)  [unwired: 12 in]
      }
      frame "--------- Motion Control ---------" {
      }
      frame "Motion: Energize Drives" {
        n125 = in-place {
          in-place-border: w416 -> [w423]
          in-place-border: [w420] -> w413
          n126 = in-place-cluster #10(w415) -> ("Motion-ControlAll.lvclass"=w422:refnum<class "Motion-ControlAll.lvclass">)
          n127 = call "Motion-Energize-Drives.vi"("error in (no error)"=w423, "Motion-ControlAll in"=w422) -> ("error out"=w420:errorcluster, "Motion-ControlAll out"=w421:refnum<class "Motion-ControlAll.lvclass">)  [unwired: 8 in]
          n128 = in-place-cluster #10("Motion-ControlAll.lvclass"=w421) -> (w414:refnum<class "Material-RunTest.lvclass">)
        }
      }
      frame "Motion: DeEnergize Drives" {
        n129 = in-place {
          in-place-border: w427 -> [w434]
          in-place-border: [w431] -> w424
          n130 = in-place-cluster #11(w426) -> ("Motion-ControlAll.lvclass"=w433:refnum<class "Motion-ControlAll.lvclass">)
          n131 = call "Motion-DeEnergize-Drives.vi"("error in (no error)"=w434, "Motion-ControlAll in"=w433) -> ("error out"=w431:errorcluster, "Motion-ControlAll out"=w432:refnum<class "Motion-ControlAll.lvclass">)  [unwired: 8 in]
          n132 = in-place-cluster #11("Motion-ControlAll.lvclass"=w432) -> (w425:refnum<class "Material-RunTest.lvclass">)
        }
      }
      frame "Motion: Find Home Position" {
        n133 = in-place {
          in-place-border: w440 -> [w447]
          in-place-border: [w444] -> w437
          n134 = in-place-cluster #12(w439) -> ("Motion-ControlAll.lvclass"=w446:refnum<class "Motion-ControlAll.lvclass">)
          n135 = call "Motion-FindHome.vi"("error in (no error)"=w447, "Motion-ControlAll in"=w446) -> ("error out"=w444:errorcluster, "Motion-ControlAll out"=w445:refnum<class "Motion-ControlAll.lvclass">)  [unwired: 8 in]
          n136 = in-place-cluster #12("Motion-ControlAll.lvclass"=w445) -> (w438:refnum<class "Material-RunTest.lvclass">)
        }
        n137 = property on="Find Home Position" class="Bool (strict)"(error in=w437, "Value"=FALSE ("Find Home Position")) -> (error out=w436:errorcluster)  [unwired: 1 in, 1 out]
      }
      frame "Motion: Close Connection" {
        n138 = in-place {
          in-place-border: w451 -> [w458]
          in-place-border: [w457] -> w448
          n139 = in-place-cluster #13(w450) -> ("Motion-ControlAll.lvclass"=w455:refnum<class "Motion-ControlAll.lvclass">)
          n140 = call "Motion-Close.vi"("error in (no error)"=w458, "Motion-ControlAll in"=w455) -> ("error out"=w457:errorcluster, "Motion-ControlAll out"=w456:refnum<class "Motion-ControlAll.lvclass">)  [unwired: 8 in]
          n141 = in-place-cluster #13("Motion-ControlAll.lvclass"=w456) -> (w449:refnum<class "Material-RunTest.lvclass">)
        }
      }
      frame "-----------Keyence Laser-------------" {
      }
      frame "Laser: Change Sampling Rate" {
        n142 = call "Material-Laser-ChangeSamplingRate.vi"("error in (no error)"=w472, "Material-RunTest in"=w471) -> ("error out"=w464:errorcluster, "Rate updated?"=w466:bool, "Material-RunTest out"=w470:refnum<class "Material-RunTest.lvclass">)  [unwired: 7 in]
        n143 = case shown="True" w466 {
          tunnel: ["" ("Add Next in Sequence") "Sequence: Zero Laser Routine\nSequence: Load Sheet" ("Add Next in Sequence")] -> w467
          tunnel: [w475 w482] -> w465
          tunnel: w464 -> [_ w482]
          frame False {
            n144 = xnode "Error Ring"() -> ("error out"=w475:errorcluster)
          }
          frame True {
          }
        }
        n145 = call "FTW-SEQ-AddNext.vi"("Add Next in Sequence"=w467, "Sequencer"=w469) -> ("Sequencer out"=w468:refnum<class "FTW-Sequencer.lvclass">)  [unwired: 2 in]
      }
    }
  }
  "error out" <- w2
  n146 = call "FTW-SEQ-Destroy.vi"("Sequencer"=w3) -> ()  [unwired: 1 in]
